vi "Touch Panel Main.vi"() -> ()   [LabVIEW 2020]
doc: "Use this template to create a Touch Panel VI."
panel:
  in  "Tab Control":T1(tab)
  in  "Scaling <Replace Me>":dbl(slide)=1.0 step=0.25 scale=0.0..10.0
  out "Data":dbl(graph)
  out "Alarm <Replace Me>":bool
  in  "Exit":bool
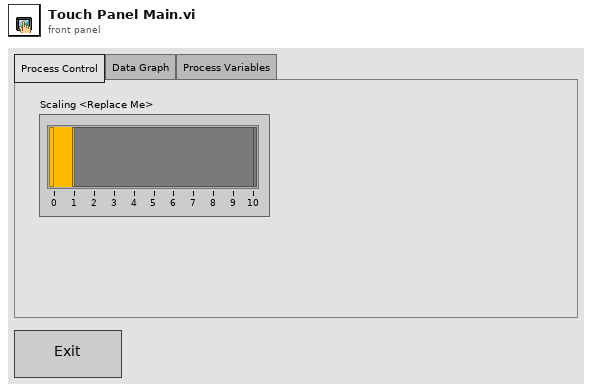
[diagram p1: front panel]
types:
  T1 = enum32{"Process Control", "Data Graph", "Process Variables"}
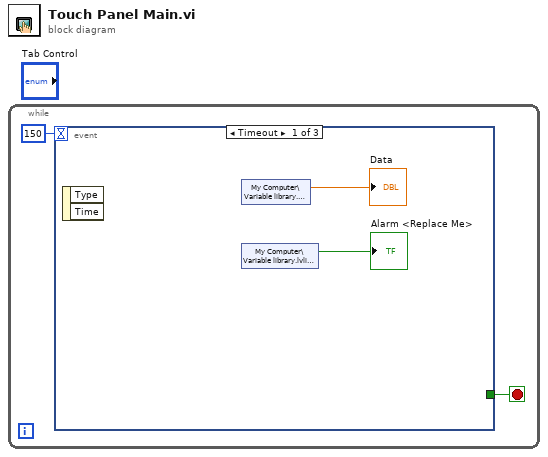
[diagram p0: block diagram]
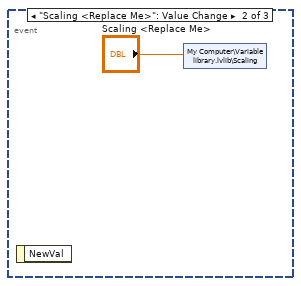
[diagram p2: hidden frame]
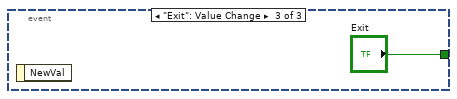
[diagram p3: hidden frame]
diagram:
  n1 = while {
    stop <- w2 stop-if-true
    n2 = event shown="[0] Timeout" {
      selector: _ -> [_ _ _]
      dyn-events: _ -> [_ _ _]
      timeout: 150 -> [_ _ _]
      tunnel: [_ _ "Exit"] -> w2
      event Timeout {
        n3 = event-data() -> ()  [unwired: 1 in, 2 out]
        n4 = shared-variable "My Computer\\Variable library.lvlib\\Data"() -> (→"Data":dbl)  [unwired: 1 in, 1 out]
        n5 = shared-variable "My Computer\\Variable library.lvlib\\Alarm"() -> (→"Alarm <Replace Me>":bool)  [unwired: 1 in, 1 out]
      }
      event "Scaling <Replace Me>": Value Change {
        n6 = event-data() -> ()  [unwired: 1 in, 1 out]
        n7 = shared-variable "My Computer\\Variable library.lvlib\\Scaling"("Scaling <Replace Me>") -> ()  [unwired: 1 in, 1 out]
      }
      event "Exit": Value Change {
        n8 = event-data() -> ()  [unwired: 1 in, 1 out]
      }
    }
  }
